vi "Action 1.vi"(8 "error in (no error)":errorcluster, 11 "Interface 3 in":refnum<class "Class 1.lvclass">) -> (0 "error out":errorcluster, 3 "Interface 3 out":refnum<class "Class 1.lvclass">)   [LabVIEW 2021, in "Untitled Library 64.lvlib" / "Class 1.lvclass"]
uses:
  Class 1.lvclass
  Class 1.lvclass/Class 1.ctl
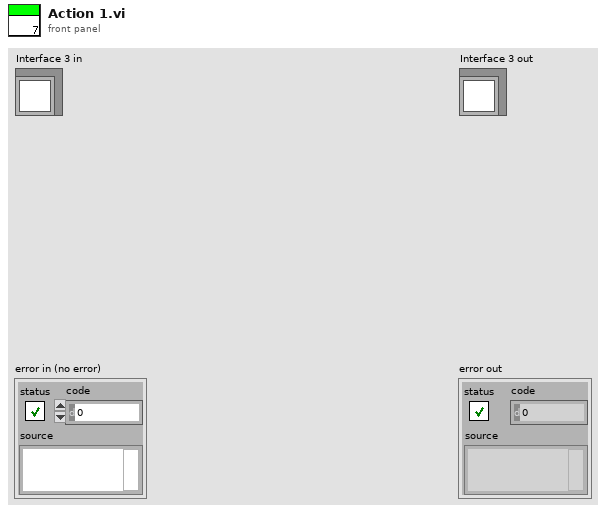
[diagram p1: front panel]
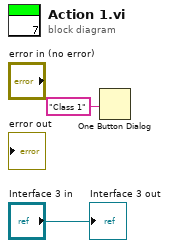
[diagram p0: block diagram]
diagram:
  n1 = One Button Dialog(message="Class 1") -> ()  [unwired: 1 in, 1 out]
  "Interface 3 out" <- "Interface 3 in"
